vi "Initialization VI.vi"(8 "error in (no error)":errorcluster, 10 "Custom XML":string, 11 "Device Item Ref in":T1 format="%.0x") -> (0 "error out":errorcluster, 3 "Device Item Ref out":T1 format="%.0x")   [LabVIEW 2023, in "Protection and Counter Addon System Explorer.lvlib"]
uses:
  Protection and Counter Addon System Explorer.lvlib
  <vilib>/NI VeriStand/Custom Device API/Custom Device Item Ref.ctl
  <vilib>/NI VeriStand/Custom Device API/Custom Device Channel.ctl
  <vilib>/NI VeriStand/Custom Device API/Custom Device Channel Type.ctl
  <vilib>/NI VeriStand/Custom Device API/Custom Device File Dependency.ctl
  <vilib>/NI VeriStand/Custom Device API/Path Specification.ctl
  <vilib>/NI VeriStand/Custom Device API/Path Type.ctl
  <vilib>/NI VeriStand/Custom Device API/Custom Device Supported Target.ctl
  Addon Shared/SubVIs/GUID Lookup.vi
  <vilib>/NI VeriStand/Custom Device API/Custom Device API.lvlib
  Addon Shared/Protection and Counter Addon Shared.lvlib
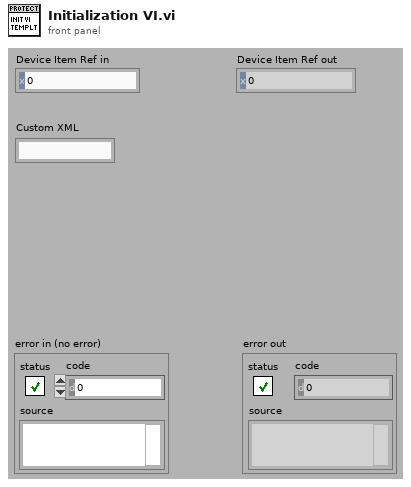
[diagram p1: front panel]
types:
  T1 = typedef "Custom Device API.lvlib/Custom Device Item Ref.ctl" = u64
  T2 = typedef "Custom Device API.lvlib/Custom Device File Dependency.ctl" = cluster{"Source":T3, "RT Destination":path, "ForceDownload?":bool, "SupportedTarget":T5, "Version":string}
  T3 = typedef "Custom Device API.lvlib/Path Specification.ctl" = cluster{"Path":path, "Type":T4}
  T4 = typedef "Custom Device API.lvlib/Path Type.ctl" = enum16{"Absolute", "To Base", "To Common Data Dir", "To Application Data Dir"}
  T5 = typedef "Custom Device API.lvlib/Custom Device Supported Target.ctl" = enum16{"All", "PharLap", "VxWorks", "Windows", "Linux_32_ARM", "Linux_x64", "PharLap & Windows", "PharLap & VxWorks", "VxWorks & Windows"}
  T6 = typedef "Custom Device API.lvlib/Custom Device Channel.ctl" = cluster{"Type":T7, "Units":string, "Default Value":dbl, "Faultable":bool, "Scalable":bool}
  T7 = typedef "Custom Device API.lvlib/Custom Device Channel Type.ctl" = enum16{"Input", "Output"}
  T8 = typedef "Protection and Counter Addon Shared.lvlib/XNET Settings.ctl" = cluster{"Database":refnum<k21>, "Cluster":refnum<k21>, "Port":string, "Baud rate [Bd]":u64, "Termination":u32, "CAN I/O Mode":u32, "FD Baud rate [Bd]":u64, "Priority":i32, "Use Legacy":bool, "FD ISO Mode":u32}
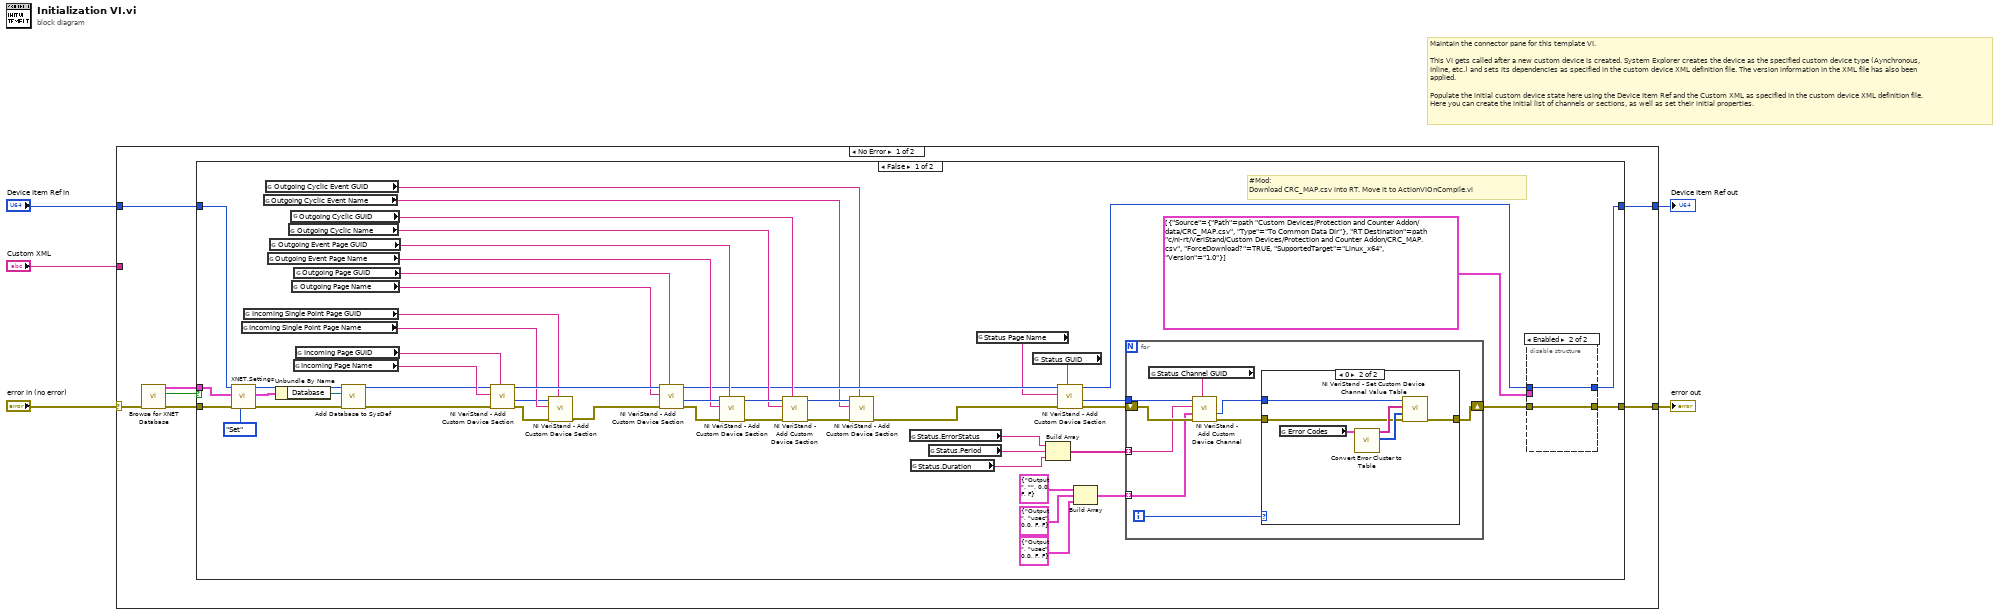
[diagram p0: block diagram]
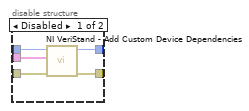
[diagram p2: hidden frame]
diagram:
  # "Maintain the connector pane for this template VI.\n\nThis VI gets called after a new custom device is created. System Explorer creates the device as the specified custom device type (Aynchronous, Inline, etc.) and sets its dependencies as specified in the custom device XML definition file. The version information in the XML file has also been applied.\n\nPopulate the initial custom device state here using the Device Item Ref and the Custom XML as specified in the custom device XML definition file. Here you can create the initial list of channels or sections, as well as set their initial properties."
  n1 = case shown="No Error" "error in (no error)" {
    selector: "error in (no error)" -> [w10 w90]
    tunnel: [w12 w90] -> w5
    tunnel: [w11 w89] -> w3
    tunnel: "Device Item Ref in" -> [w8 w89]
    tunnel: "Custom XML" -> [_ _]
    frame No Error {
      n2 = call "Browse for XNET Database.vi"("error in (no error)"=w10) -> ("error out"=w9:errorcluster, "Cancel Out"=w7:bool, "XNET Settings"=w6:T8)  [unwired: 8 in]
      n3 = case shown="False" w7 {
        tunnel: [w16 w88] -> w12
        tunnel: [w14 w87] -> w11
        tunnel: w9 -> [w56 w88]
        tunnel: w8 -> [w54 w87]
        tunnel: w6 -> [w52 _]
        frame False {
          # "#Mod:\nDownload CRC_MAP.csv into RT. Move it to ActionVIOnCompile.vi"
          n4 = call "XNET.Settings.vi"("Action"=enum8{"Get", "Set"}."Set", "error in (no error)"=w56, "XNET Settings"=w52, "Parent Ref in"=w54) -> ("error out"=w55:errorcluster, "XNET Settings"=w51:T8, "Item Ref out"=w53:T1)  [unwired: 5 in]
          n5 = global read "GUID Lookup.vi" "Incoming Single Point Page Name"() -> (w38:string)
          n6 = global read "GUID Lookup.vi" "Incoming Single Point Page GUID"() -> (w39:string)
          n7 = global read "GUID Lookup.vi" "Outgoing Cyclic Event Name"() -> (w24:string)
          n8 = global read "GUID Lookup.vi" "Outgoing Cyclic Event GUID"() -> (w25:string)
          n9 = global read "GUID Lookup.vi" "Outgoing Event Page Name"() -> (w43:string)
          n10 = global read "GUID Lookup.vi" "Outgoing Event Page GUID"() -> (w44:string)
          n11 = Unbundle By Name(w51) -> ("Database"=w50:refnum<k21>)
          n12 = global read "GUID Lookup.vi" "Outgoing Cyclic Name"() -> (w41:string)
          n13 = global read "GUID Lookup.vi" "Outgoing Cyclic GUID"() -> (w42:string)
          n14 = global read "GUID Lookup.vi" "Outgoing Page Name"() -> (w60:string)
          n15 = global read "GUID Lookup.vi" "Incoming Page Name"() -> (w59:string)
          n16 = global read "GUID Lookup.vi" "Outgoing Page GUID"() -> (w61:string)
          n17 = global read "GUID Lookup.vi" "Incoming Page GUID"() -> (w63:string)
          n18 = call "Add Database to SysDef.vi"("error in"=w55, "DB Alias"=w50, "Item Ref in"=w53) -> ("error out"=w58:errorcluster, "Item Ref out"=w57:T1)  [unwired: 7 in]
          n19 = call <vilib>:"NI VeriStand - Add Custom Device Section.vi"("GUID (Default Section)"=w63, "error in (no error)"=w58, "Section Name"=w59, "Parent Ref in"=w57) -> ("error out"=w18:errorcluster, "Section Ptr"=w19:T1, "Parent Ref out"=w62:T1)  [unwired: 4 in, 1 out]
          n20 = call <vilib>:"NI VeriStand - Add Custom Device Section.vi"("GUID (Default Section)"=w39, "error in (no error)"=w18, "Section Name"=w38, "Parent Ref in"=w19) -> ("error out"=w40:errorcluster)  [unwired: 4 in, 3 out]
          n21 = call <vilib>:"NI VeriStand - Add Custom Device Section.vi"("GUID (Default Section)"=w61, "error in (no error)"=w40, "Section Name"=w60, "Parent Ref in"=w62) -> ("error out"=w46:errorcluster, "Section Ptr"=w48:T1, "Parent Ref out"=w35:T1)  [unwired: 4 in, 1 out]
          n22 = call <vilib>:"NI VeriStand - Add Custom Device Section.vi"("GUID (Default Section)"=w44, "error in (no error)"=w46, "Section Name"=w43, "Parent Ref in"=w48) -> ("error out"=w47:errorcluster, "Parent Ref out"=w45:T1)  [unwired: 4 in, 2 out]
          n23 = call <vilib>:"NI VeriStand - Add Custom Device Section.vi"("GUID (Default Section)"=w42, "error in (no error)"=w47, "Section Name"=w41, "Parent Ref in"=w45) -> ("error out"=w27:errorcluster, "Parent Ref out"=w28:T1)  [unwired: 4 in, 2 out]
          n24 = call <vilib>:"NI VeriStand - Add Custom Device Section.vi"("GUID (Default Section)"=w25, "error in (no error)"=w27, "Section Name"=w24, "Parent Ref in"=w28) -> ("error out"=w26:errorcluster)  [unwired: 4 in, 3 out]
          n25 = global read "GUID Lookup.vi" "Status.ErrorStatus"() -> (w34:string)
          n26 = global read "GUID Lookup.vi" "Status.Duration"() -> (w32:string)
          n27 = global read "GUID Lookup.vi" "Status.Period"() -> (w33:string)
          n28 = global read "GUID Lookup.vi" "Status Page Name"() -> (w29:string)
          n29 = global read "GUID Lookup.vi" "Status GUID"() -> (w30:string)
          n30 = Build Array(w34, w33, w32) -> (w31:string[])
          n31 = call <vilib>:"NI VeriStand - Add Custom Device Section.vi"("GUID (Default Section)"=w30, "error in (no error)"=w26, "Section Name"=w29, "Parent Ref in"=w35) -> ("error out"=w36:errorcluster, "Section Ptr"=w37:T1, "Parent Ref out"=w15:T1)  [unwired: 4 in, 1 out]
          n32 = Build Array(T6 {"Type"=enum."Output", "Units"="", "Default Value"=0.0, "Faultable"=FALSE, "Scalable"=FALSE} ("Channel"), T6 {"Type"=enum."Output", "Units"="usec", "Default Value"=0.0, "Faultable"=FALSE, "Scalable"=FALSE} ("Channel"), T6 {"Type"=enum."Output", "Units"="usec", "Default Value"=0.0, "Faultable"=FALSE, "Scalable"=FALSE} ("Channel")) -> (w20:T6[])
          n33 = for {
            tunnel: w37 -> [w79]
            shift-right: [w72] -> w17
            shift-left: w36 -> [w78]
            tunnel: w31 -> [w76] mode=indexing
            tunnel: w20 -> [w75] mode=indexing
            i -> [w74]
            n34 = global read "GUID Lookup.vi" "Status Channel GUID"() -> (w77:string)
            n35 = call <vilib>:"NI VeriStand - Add Custom Device Channel.vi"("GUID (Default Channel)"=w77, "error in (no error)"=w78, "Channel"=w75, "Channel Name"=w76, "Parent Ref in"=w79) -> ("error out"=w73:errorcluster, "Channel Ref"=w71:T1)  [unwired: 3 in, 2 out]
            n36 = case shown="0" w74 {
              tunnel: w71 -> [_ w85]
              tunnel: w73 -> [w80 w82]
              tunnel: [w80 w81] -> w72
              frame Default {
              }
              frame 0 {
                n37 = global read "GUID Lookup.vi" "Error Codes"() -> (w86:cluster{"number":i32, "trimmed string":string}[])
                n38 = call "Convert Error Cluster to Table.vi"("Error Codes"=w86) -> ("Code"=w83:i32[], "String"=w84:string[])  [unwired: 9 in]
                n39 = call <vilib>:"NI VeriStand - Set Custom Device Channel Value Table.vi"("error in (no error)"=w82, "Values"=w83, "Names"=w84, "Channel Ref in"=w85) -> ("error out"=w81:errorcluster)  [unwired: 6 in, 1 out]
              }
            }
          }
          n40 = disable-structure shown="Enabled" {
            disable-tunnel: w17 -> [w68 w69]
            disable-tunnel: [w67 w69] -> w16
            disable-tunnel: w15 -> [w66 w70]
            disable-tunnel: [w65 w70] -> w14
            disable-tunnel: T2[] [{"Source"={"Path"=path "Custom Devices/Protection and Counter Addon/data/CRC_MAP.csv", "Type"=enum."To Common Data Dir"}, "RT Destination"=path "c:/ni-rt/VeriStand/Custom Devices/Protection and Counter Addon/CRC_MAP.csv", "ForceDownload?"=TRUE, "SupportedTarget"=enum."Linux_x64", "Version"="1.0"}] ("Dependencies") -> [w64 _]
            frame Disabled {
              n41 = call <vilib>:"NI VeriStand - Add Custom Device Dependencies.vi"("error in (no error)"=w68, "Dependencies"=w64, "Device Ref in"=w66) -> ("error out"=w67:errorcluster, "Device Ref out"=w65:T1)  [unwired: 7 in]
            }
            frame Enabled {
            }
          }
        }
        frame True {
        }
      }
    }
    frame Error {
    }
  }
  "error out" <- w5
  "Device Item Ref out" <- w3
